vi "Periodic Tasks AUTO.vi"(8 "error in":errorcluster) -> ()   [LabVIEW 2013]
doc: "This VI runs in parallel to other tasks. It can contain as many user-defined periodic loops as you need. These can carry out PID or other sorts of timed response."
uses:
  <vilib>/Rock Robotics/SystemInterfaces/Utilities/FPGA_UtilitiesLED Source.ctl
  <vilib>/Rock Robotics/SystemInterfaces/Utilities/FPGA_UtilitiesLED State.ctl
  <vilib>/Rock Robotics/WPI/Relay/WPI_RelayValue.ctl
  <vilib>/Rock Robotics/WPI/DriverStation/DriverStationLCD/WPI_DriverStationLCDLCDLine.ctl
  <vilib>/Rock Robotics/WPI/Solenoid/WPI_SolenoidValue.ctl
  <vilib>/Rock Robotics/WPI/SafetyOutput/WPI_SafetyOutputConfigMenu.ctl
  Begin/Global Refnums.vi
  <vilib>/Rock Robotics/WPI/Solenoid/WPI_SolenoidSetEnum.vi
  <vilib>/Rock Robotics/WPI/Joystick/WPI_JoystickGetSetRefNum.vi
  <vilib>/Rock Robotics/WPI/Compressor/WPI_CompressorGetSetRefNum.vi
  Begin/Robot Global Data.vi
  Begin/Global Variables.vi
panel:
  out "Arm":string
  out "Shooter":string
  out "Winch":string
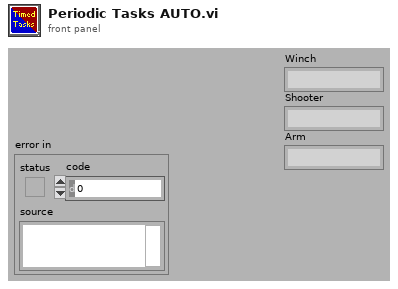
[diagram p1: front panel]
types:
  T1 = typedef "WPI_DriverStationLCDLCDLine.ctl" = enum16{"Main - Line 1", "User - Line 2", "User - Line 3", "User - Line 4", "User - Line 5", "User - Line 6"}
  T2 = typedef "WPI_CompressorDevRef.ctl" = cluster{"DevStatus":errorcluster, "DigitalInputDevRef":T3, "RelayDevRef":T6}
  T3 = typedef "WPI_DigitalInputDevRef.ctl" = cluster{"DevStatus":errorcluster, "DIO Channel":T4, "Digital Module":T5}
  T4 = typedef "FPGA_DIOChannel.ctl" = enum8{"DIO 1", "DIO 2", "DIO 3", "DIO 4", "DIO 5", "DIO 6", "DIO 7", "DIO 8", "DIO 9", "DIO 10", "DIO 11", "DIO 12", "DIO 13", "DIO 14", "Invalid"}
  T5 = typedef "FPGA_TypedefDigitalModule.ctl" = enum16{"Digital Module 1", "Digital Module 2"}
  T6 = typedef "WPI_RelayDevRef.ctl" = cluster{"DevStatus":errorcluster, "Relay Channel":T7, "Digital Module":T5, "Relay Direction":T8}
  T7 = typedef "FPGA_DIORelayChannel.ctl" = enum8{"Relay 1", "Relay 2", "Relay 3", "Relay 4", "Relay 5", "Relay 6", "Relay 7", "Relay 8", "Invalid"}
  T8 = typedef "WPI_RelayDirection.ctl" = enum16{"Both directions", "Forward only", "Reverse only"}
  T9 = typedef "WPI_RelayValue.ctl" = enum16{"Off", "On", "Forward", "Reverse"}
  T10 = typedef "WPI_SafetyOutputConfigMenu.ctl" = enum16{"Enable", "Disable"}
  T11 = typedef "WPI_SolenoidValue.ctl" = enum16{"Off", "On", "Forward", "Reverse"}
  T12 = typedef "WPI_SolenoidDevRef.ctl" = cluster{"DevStatus":errorcluster, "Solenoid Module":T13, "Forward Solenoid Channel":T14, "Reverse Solenoid Channel":T14}
  T13 = typedef "FPGA_TypedefSolenoidModule.ctl" = enum16{"Solenoid Module 1", "Solenoid Module 2"}
  T14 = typedef "WPI_SolenoidChannel.ctl" = enum8{"Solenoid 1", "Solenoid 2", "Solenoid 3", "Solenoid 4", "Solenoid 5", "Solenoid 6", "Solenoid 7", "Solenoid 8", "Invalid"}
  T15 = typedef "WPI_JoystickDevRef.ctl" = cluster{"Device":T16}
  T16 = typedef "WPI_JoystickDeviceEnum.ctl" = enum16{"USB 1", "USB 2", "USB 3", "USB 4", "Kinect 1", "Kinect 2"}
  T17 = typedef "WPI_JoystickButtonState.ctl" = cluster{"Button 1":bool, "Button 2":bool, "Button 3":bool, "Button 4":bool, "Button 5":bool, "Button 6":bool, "Button 7":bool, "Button 8":bool, "Button 9":bool, "Button 10":bool, "Button 11":bool, "Button 12":bool}
  T18 = typedef "WPI_EncoderDevRef.ctl" = cluster{"DevStatus":errorcluster, "EncoderIndex":T19, "CounterIndex":T20, "DistancePerCount":dbl, "Decoding Type":T21}
  T19 = typedef "FPGA_EncoderIdx.ctl" = enum8{"Enc 0", "Enc 1", "Enc 2", "Enc 3", "Invalid"}
  T20 = typedef "FPGA_CounterCtrSystemIndex.ctl" = enum8{"Ctr 0", "Ctr 1", "Ctr 2", "Ctr 3", "Ctr 4", "Ctr 5", "Ctr 6", "Ctr 7", "Invalid"}
  T21 = typedef "WPI_EncoderType.ctl" = enum16{"1x", "2x", "4x"}
  T22 = typedef "FPGA_UtilitiesLED State.ctl" = enum16{"Off", "On", "Toggle"}
  T23 = typedef "FPGA_UtilitiesLED Source.ctl" = enum16{"User LED", "FPGA LED"}
  T24 = typedef "WPI_MotorControlDeviceRef.ctl" = cluster{"DeviceStatus":errorcluster, "Type":enum16{"PWM", "CAN"}, "PWM":cluster{"Digital Module":T5, "PWM Channel":T25, "DeadBand":T26}, "CAN":cluster{"Device Number":u8, "Control Mode":T27, "Semaphore":T28, "Max Vout":dbl}, "Invert":bool, "TransformRef":T29, "InvTransformRef":T29}
  T25 = typedef "FPGA_DIOPWMChannel.ctl" = enum8{"PWM 1", "PWM 2", "PWM 3", "PWM 4", "PWM 5", "PWM 6", "PWM 7", "PWM 8", "PWM 9", "PWM 10", "Invalid"}
  T26 = typedef "WPI_PWMDeadband.ctl" = cluster{"Name":string, "maxPositivePwm":i32, "minPositivePwm":i32, "centerPwm":i32, "maxNegativePwm":i32, "minNegativePwm":i32, "angularRange":u16}
  T27 = typedef "WPI_CANJaguar_ControlMode.ctl" = enum8{"Percent VBus", "Current", "Speed", "Position", "Voltage"}
  T28 = typedef "Semaphore RefNum" = refnum<k1>
  T29 = typedef "WPI_PWMTransform_ConPane.ctl" = refnum<vi>
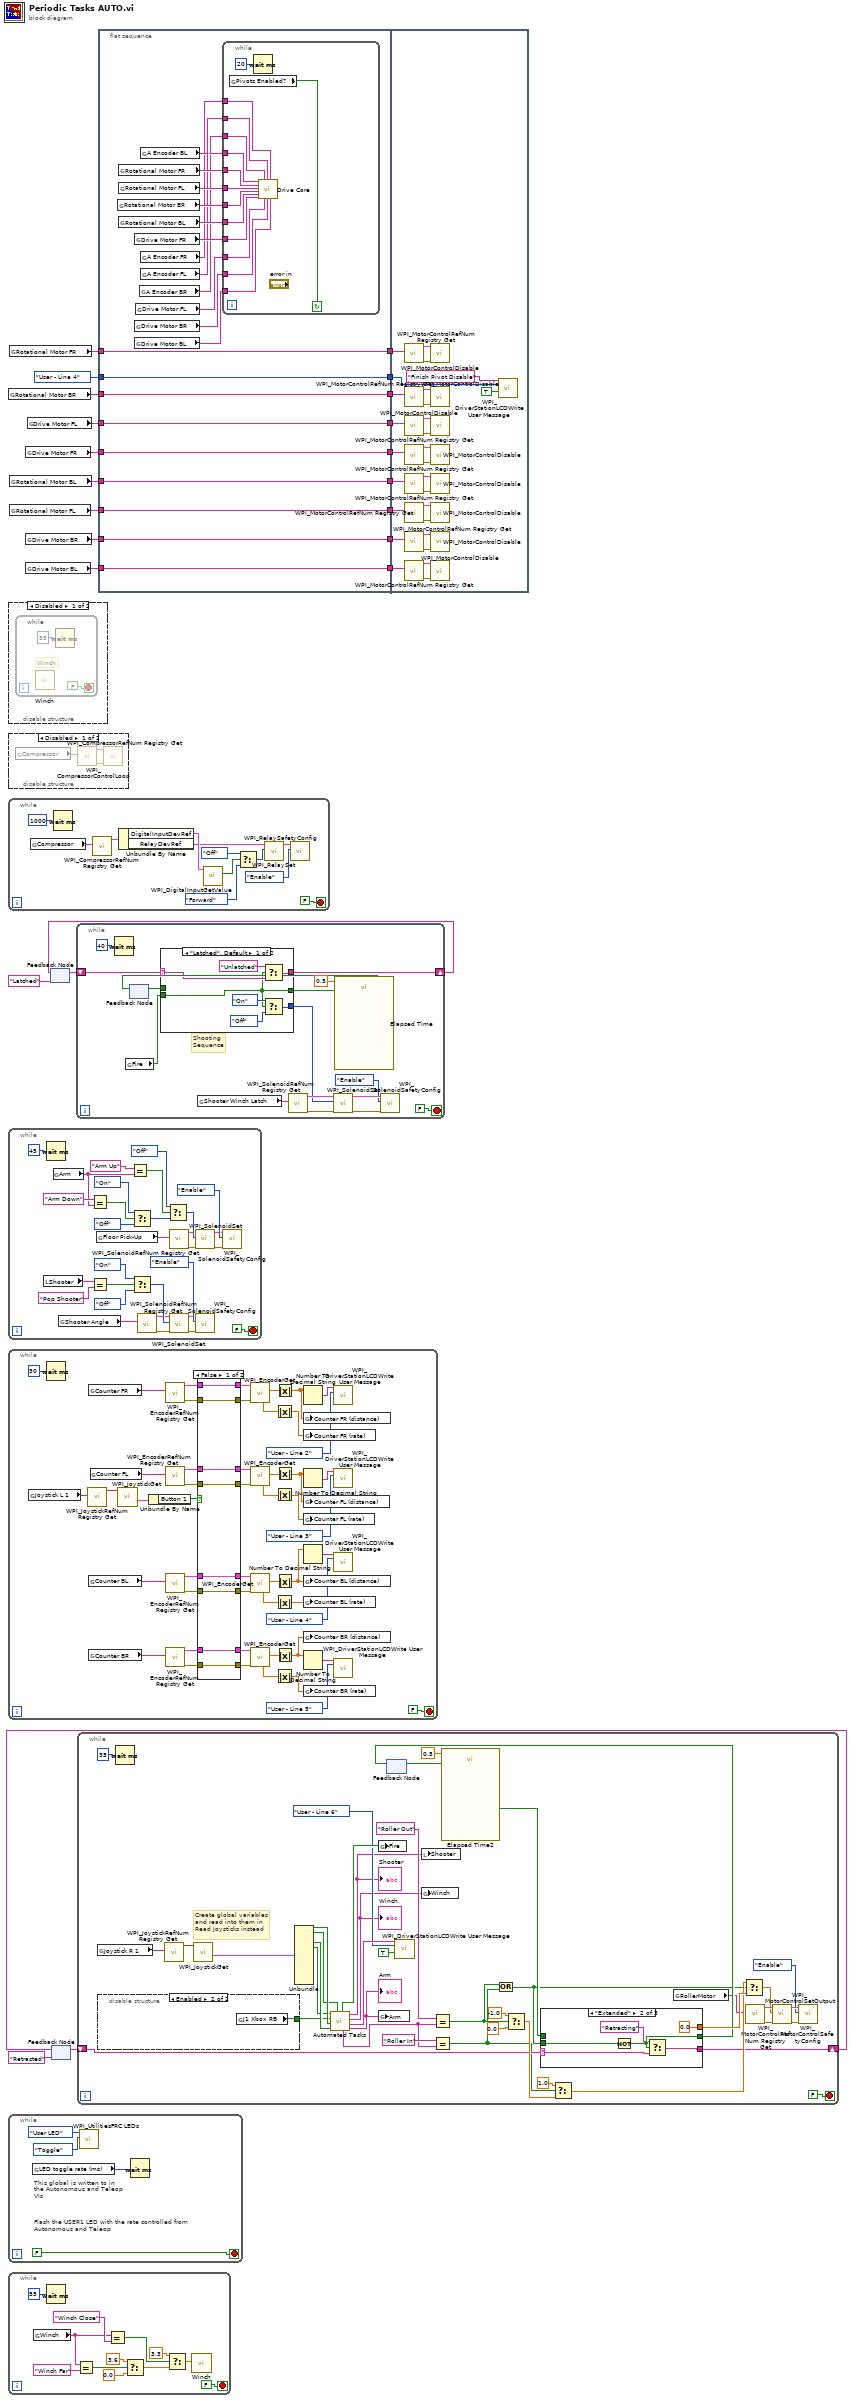
[diagram p0: block diagram]
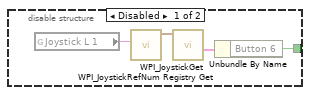
[diagram p3: hidden frame]
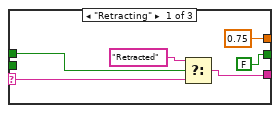
[diagram p4: hidden frame]
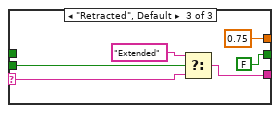
[diagram p5: hidden frame]
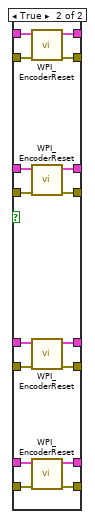
[diagram p6: hidden frame]
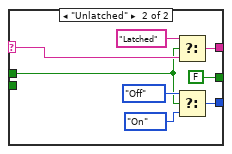
[diagram p7: hidden frame]
diagram:
  n1 = global read "Global Refnums.vi" "Rotational Motor BR"() -> (w22:string)
  n2 = disable-structure shown="Disabled" {
    frame Disabled {
      n3 = while {
        stop <- FALSE stop-if-true
        # "Winch"
        n4 = call "Winch.vi"() -> ()  [unwired: 12 in]
        n5 = Wait (ms)(milliseconds to wait=u32 35) -> ()  [unwired: 1 out]
      }
    }
    frame Enabled {
    }
  }
  n6 = disable-structure shown="Disabled" {
    frame Disabled {
      n7 = global read "Global Refnums.vi" "Compressor"() -> (w29:string)
      n8 = call <vilib>:"WPI_CompressorRefNum Registry Get.vi"("refnum name"=w29) -> ("error out"=w28:errorcluster, "CompressorDevRef"=w27:T2)  [unwired: 9 in]
      n9 = call <vilib>:"WPI_CompressorControlLoop.vi"("error in (no error)"=w28, "CompressorDevRef"=w27) -> ()  [unwired: 10 in]
    }
    frame Enabled {
    }
  }
  n10 = while {
    stop <- FALSE stop-if-true
    n11 = global read "Global Refnums.vi" "Compressor"() -> (w39:string)
    n12 = Wait (ms)(milliseconds to wait=1000) -> ()  [unwired: 1 out]
    n13 = call <vilib>:"WPI_CompressorRefNum Registry Get.vi"("refnum name"=w39) -> ("CompressorDevRef"=w38:T2)  [unwired: 9 in, 1 out]
    n14 = Unbundle By Name(w38) -> ("DigitalInputDevRef"=w37:T3, "RelayDevRef"=w36:T6)
    n15 = call <vilib>:"WPI_DigitalInputGetValue.vi"("DigitalInputDevRef"=w37) -> ("Value"=w33:bool)  [unwired: 8 in, 2 out]
    n16 = Select(t=WPI_RelayValue."Off" ("RelayValue"), s=w33, f=WPI_RelayValue."Forward" ("RelayValue")) -> (s? t:f=w32:T9)
    n17 = call <vilib>:"WPI_RelaySet.vi"("RelayValue"=w32, "RelayDevRef"=w36) -> ("RelayDevRef"=w35:T6)  [unwired: 8 in, 1 out]
    n18 = call <vilib>:"WPI_RelaySafetyConfig.vi"("mode"=WPI_SafetyOutputConfigMenu."Enable", "RelayDevRef"=w35) -> ()  [unwired: 8 in, 2 out]
  }
  n19 = while {
    stop <- FALSE stop-if-true
    n20 = local read "Shooter"() -> (w59:string)
    n21 = Wait (ms)(milliseconds to wait=u32 45) -> ()  [unwired: 1 out]
    n22 = global read "Global Refnums.vi" "Arm"() -> (w42:string)
    n23 = global read "Global Refnums.vi" "Shooter Angle"() -> (w70:string)
    n24 = Equal?(x="Arm Down", y=w42) -> (x = y?=w44:bool)
    n25 = Equal?(x=w59, y="Pop Shooter") -> (x = y?=w60:bool)
    n26 = global read "Global Refnums.vi" "Floor Pick-Up"() -> (w54:string)
    n27 = Equal?(x="Arm Up", y=w42) -> (x = y?=w56:bool)
    n28 = Select(t=WPI_SolenoidValue."On" ("Value"), s=w44, f=WPI_SolenoidValue."Off" ("Value")) -> (s? t:f=w43:T11)
    n29 = Select(t=WPI_SolenoidValue."On" ("Value"), s=w60, f=WPI_SolenoidValue."Off" ("Value")) -> (s? t:f=w69:T11)
    n30 = call <vilib>:"WPI_SolenoidRefNum Registry Get.vi"("refnum name"=w70) -> ("error out"=w62:errorcluster, "SolenoidDevRef"=w63:T12)  [unwired: 9 in]
    n31 = Select(t=WPI_SolenoidValue."Off" ("Value"), s=w56, f=w43) -> (s? t:f=w57:T11)
    n32 = call <vilib>:"WPI_SolenoidRefNum Registry Get.vi"("refnum name"=w54) -> ("error out"=w49:errorcluster, "SolenoidDevRef"=w50:T12)  [unwired: 9 in]
    n33 = call-poly <vilib>:"WPI_SolenoidSet.vi"("error in (no error)"=w62, "Value"=w69, "SolenoidDevRef"=w63) -> ("error out"=w65:errorcluster, "SolenoidDevRef"=w64:T12)  [unwired: 7 in]
    n34 = call-poly <vilib>:"WPI_SolenoidSet.vi"("error in (no error)"=w49, "Value"=w57, "SolenoidDevRef"=w50) -> ("error out"=w52:errorcluster, "SolenoidDevRef"=w51:T12)  [unwired: 7 in]
    n35 = call <vilib>:"WPI_SolenoidSafetyConfig.vi"("error in (no error)"=w65, "mode"=WPI_SafetyOutputConfigMenu."Enable", "SolenoidDevRef"=w64) -> ()  [unwired: 7 in, 2 out]
    n36 = call <vilib>:"WPI_SolenoidSafetyConfig.vi"("error in (no error)"=w52, "mode"=WPI_SafetyOutputConfigMenu."Enable", "SolenoidDevRef"=w51) -> ()  [unwired: 7 in, 2 out]
  }
  n37 = while {
    stop <- FALSE stop-if-true
    n38 = global read "Global Refnums.vi" "Joystick L 1"() -> (w118:string)
    n39 = Wait (ms)(milliseconds to wait=u32 30) -> ()  [unwired: 1 out]
    n40 = call <vilib>:"WPI_JoystickRefNum Registry Get.vi"("refnum name"=w118) -> ("JoystickDevRef"=w119:T15)  [unwired: 9 in, 1 out]
    n41 = global read "Global Refnums.vi" "Counter FR"() -> (w82:string)
    n42 = global read "Global Refnums.vi" "Counter BL"() -> (w83:string)
    n43 = global read "Global Refnums.vi" "Counter BR"() -> (w80:string)
    n44 = global read "Global Refnums.vi" "Counter FL"() -> (w81:string)
    n45 = call <vilib>:"WPI_JoystickGet.vi"("JoystickDevRef"=w119) -> ("Buttons"=w117:T17)  [unwired: 4 in, 2 out]
    n46 = Unbundle By Name(w117) -> ("Button 1"=w116:bool)
    n47 = call <vilib>:"WPI_EncoderRefNum Registry Get.vi"("refnum name"=w82) -> ("error out"=w100:errorcluster, "EncoderDevRef"=w103:T18)  [unwired: 9 in]
    n48 = call <vilib>:"WPI_EncoderRefNum Registry Get.vi"("refnum name"=w81) -> ("error out"=w105:errorcluster, "EncoderDevRef"=w106:T18)  [unwired: 9 in]
    n49 = call <vilib>:"WPI_EncoderRefNum Registry Get.vi"("refnum name"=w83) -> ("error out"=w110:errorcluster, "EncoderDevRef"=w111:T18)  [unwired: 9 in]
    n50 = call <vilib>:"WPI_EncoderRefNum Registry Get.vi"("refnum name"=w80) -> ("error out"=w108:errorcluster, "EncoderDevRef"=w109:T18)  [unwired: 9 in]
    n51 = case shown="False" w116 {
      tunnel: w109 -> [w126 w145]
      tunnel: [w126 w144] -> w114
      tunnel: [w128 w143] -> w115
      tunnel: w108 -> [w128 w142]
      tunnel: [w127 w141] -> w113
      tunnel: [w129 w140] -> w112
      tunnel: w111 -> [w127 w139]
      tunnel: w110 -> [w129 w138]
      tunnel: [w125 w130] -> w107
      tunnel: w106 -> [w125 w137]
      tunnel: w105 -> [w124 w136]
      tunnel: [w124 w131] -> w104
      tunnel: w103 -> [w123 w135]
      tunnel: [w123 w132] -> w102
      tunnel: [w122 w133] -> w101
      tunnel: w100 -> [w122 w134]
      frame False {
      }
      frame True {
        n52 = call <vilib>:"WPI_EncoderReset.vi"("error in (no error)"=w134, "EncoderDevRef"=w135) -> ("error out"=w133:errorcluster, "EncoderDevRef"=w132:T18)  [unwired: 8 in]
        n53 = call <vilib>:"WPI_EncoderReset.vi"("error in (no error)"=w136, "EncoderDevRef"=w137) -> ("error out"=w131:errorcluster, "EncoderDevRef"=w130:T18)  [unwired: 8 in]
        n54 = call <vilib>:"WPI_EncoderReset.vi"("error in (no error)"=w138, "EncoderDevRef"=w139) -> ("error out"=w140:errorcluster, "EncoderDevRef"=w141:T18)  [unwired: 8 in]
        n55 = call <vilib>:"WPI_EncoderReset.vi"("error in (no error)"=w142, "EncoderDevRef"=w145) -> ("error out"=w143:errorcluster, "EncoderDevRef"=w144:T18)  [unwired: 8 in]
      }
    }
    n56 = call <vilib>:"WPI_EncoderGet.vi"("error in (no error)"=w101, "EncoderDevRef"=w102) -> ("Distance"=w97:dbl, "Rate"=w93:dbl)  [unwired: 4 in, 4 out]
    n57 = call <vilib>:"WPI_EncoderGet.vi"("error in (no error)"=w104, "EncoderDevRef"=w107) -> ("Distance"=w99:dbl, "Rate"=w95:dbl)  [unwired: 4 in, 4 out]
    n58 = call <vilib>:"WPI_EncoderGet.vi"("error in (no error)"=w112, "EncoderDevRef"=w113) -> ("Distance"=w98:dbl, "Rate"=w94:dbl)  [unwired: 4 in, 4 out]
    n59 = call <vilib>:"WPI_EncoderGet.vi"("error in (no error)"=w115, "EncoderDevRef"=w114) -> ("Distance"=w96:dbl, "Rate"=w92:dbl)  [unwired: 4 in, 4 out]
    n60 = Absolute Value(x=w93) -> (abs(x)=w78:dbl)
    n61 = Absolute Value(x=w95) -> (abs(x)=w76:dbl)
    n62 = Absolute Value(x=w94) -> (abs(x)=w74:dbl)
    n63 = Absolute Value(x=w92) -> (abs(x)=w72:dbl)
    n64 = Absolute Value(x=w97) -> (abs(x)=w79:dbl)
    n65 = Absolute Value(x=w99) -> (abs(x)=w77:dbl)
    n66 = Absolute Value(x=w98) -> (abs(x)=w75:dbl)
    n67 = Absolute Value(x=w96) -> (abs(x)=w73:dbl)
    n68 = Number To Decimal String(number=w79) -> (decimal integer string=w90:string)  [unwired: 1 in]
    n69 = global write "Global Refnums.vi" "Counter FR (distance)"(w79) -> ()
    n70 = global write "Global Refnums.vi" "Counter FR (rate)"(w78) -> ()
    n71 = Number To Decimal String(number=w77) -> (decimal integer string=w89:string)  [unwired: 1 in]
    n72 = global write "Global Refnums.vi" "Counter FL (distance)"(w77) -> ()
    n73 = global write "Global Refnums.vi" "Counter FL (rate)"(w76) -> ()
    n74 = Number To Decimal String(number=w75) -> (decimal integer string=w88:string)  [unwired: 1 in]
    n75 = global write "Global Refnums.vi" "Counter BL (distance)"(w75) -> ()
    n76 = global write "Global Refnums.vi" "Counter BL (rate)"(w74) -> ()
    n77 = global write "Global Refnums.vi" "Counter BR (distance)"(w73) -> ()
    n78 = Number To Decimal String(number=w73) -> (decimal integer string=w91:string)  [unwired: 1 in]
    n79 = global write "Global Refnums.vi" "Counter BR (rate)"(w72) -> ()
    n80 = call <vilib>:"WPI_DriverStationLCDWrite User Message.vi"("line text"=w90, "line"=WPI_DriverStationLCDLCDLine."User - Line 2") -> ()  [unwired: 13 in, 1 out]
    n81 = call <vilib>:"WPI_DriverStationLCDWrite User Message.vi"("line text"=w89, "line"=WPI_DriverStationLCDLCDLine."User - Line 3") -> ()  [unwired: 13 in, 1 out]
    n82 = call <vilib>:"WPI_DriverStationLCDWrite User Message.vi"("line text"=w88, "line"=WPI_DriverStationLCDLCDLine."User - Line 4") -> ()  [unwired: 13 in, 1 out]
    n83 = call <vilib>:"WPI_DriverStationLCDWrite User Message.vi"("line text"=w91, "line"=WPI_DriverStationLCDLCDLine."User - Line 5") -> ()  [unwired: 13 in, 1 out]
  }
  n84 = while {
    stop <- FALSE stop-if-true
    # "This global is written to in the Autonomous and Teleop VIs"
    # "Flash the USER1 LED with the rate controlled from Autonomous and Teleop"
    n85 = global read "Robot Global Data.vi" "LED toggle rate (ms)"() -> (w146:u32)
    n86 = call <vilib>:"WPI_UtilitiesFRC LEDs.vi"("State"=FPGA_UtilitiesLED_State."Toggle", "LED Type"=FPGA_UtilitiesLED_Source."User LED") -> ()  [unwired: 1 in, 9 out]
    n87 = Wait (ms)(milliseconds to wait=w146) -> ()  [unwired: 1 out]
  }
  n88 = while {
    stop <- FALSE stop-if-true
    n89 = global read "Global Refnums.vi" "Winch"() -> (w150:string)
    n90 = Wait (ms)(milliseconds to wait=u32 55) -> ()  [unwired: 1 out]
    n91 = Equal?(x=w150, y="Winch Far") -> (x = y?=w156:bool)
    n92 = Equal?(x=w150, y="Winch Close") -> (x = y?=w154:bool)
    n93 = Select(t=3.6, s=w156, f=0.0) -> (s? t:f=w158:dbl)
    n94 = Select(t=3.3, s=w154, f=w158) -> (s? t:f=w159:dbl)
    n95 = call "Winch.vi"("setpoint"=w159) -> ()  [unwired: 11 in]
  }
  n96 = global read "Global Refnums.vi" "Rotational Motor FR"() -> (w24:string)
  n97 = global read "Global Refnums.vi" "Rotational Motor BL"() -> (w21:string)
  n98 = global read "Global Refnums.vi" "Rotational Motor FL"() -> (w23:string)
  n99 = global read "Global Refnums.vi" "Drive Motor FR"() -> (w20:string)
  n100 = global read "Global Refnums.vi" "Drive Motor BR"() -> (w18:string)
  n101 = global read "Global Refnums.vi" "Drive Motor BL"() -> (w17:string)
  n102 = global read "Global Refnums.vi" "Drive Motor FL"() -> (w19:string)
  n103 = feedback #1("Latched") -> (w5:string)
  n104 = feedback #2("Retracted") -> (w2:string)
  n105 = while {
    shift-right: [w171] -> w6
    shift-left: w5 -> [w170]
    stop <- FALSE stop-if-true
    # "Shooting\nSequence"
    n106 = Wait (ms)(milliseconds to wait=u32 40) -> ()  [unwired: 1 out]
    n107 = global read "Global Variables.vi" "Fire"() -> (w169:bool)
    n108 = feedback #3() -> (w165:bool)  [unwired: 1 in]
    n109 = case shown="\"Latched\", Default" w170 {
      selector: w170 -> [w183 w191]
      tunnel: [w182 w190] -> w171
      tunnel: w169 -> [w178 _]
      tunnel: [w179 w187] -> w168
      tunnel: [w178 FALSE] -> w167
      tunnel: w165 -> [_ w186]
      frame "Latched", Default {
        n110 = Select(t="Unlatched", s=w178, f=w183) -> (s? t:f=w182:string)
        n111 = Select(t=WPI_SolenoidValue."On" ("Value"), s=w178, f=WPI_SolenoidValue."Off" ("Value")) -> (s? t:f=w179:T11)
      }
      frame "Unlatched" {
        n112 = Select(t="Latched", s=w186, f=w191) -> (s? t:f=w190:string)
        n113 = Select(t=WPI_SolenoidValue."Off" ("Value"), s=w186, f=WPI_SolenoidValue."On" ("Value")) -> (s? t:f=w187:T11)
      }
    }
    n114 = global read "Global Refnums.vi" "Shooter Winch Latch"() -> (w177:string)
    n115 = call <vilib>:"WPI_SolenoidRefNum Registry Get.vi"("refnum name"=w177) -> ("error out"=w176:errorcluster, "SolenoidDevRef"=w175:T12)  [unwired: 9 in]
    n116 = call-poly <vilib>:"WPI_SolenoidSet.vi"("error in (no error)"=w176, "Value"=w168, "SolenoidDevRef"=w175) -> ("error out"=w174:errorcluster, "SolenoidDevRef"=w173:T12)  [unwired: 7 in]
    n117 = call "Elapsed Time"("Time Target (s)"=0.5, "Reset"=w167) -> ("Time has Elapsed"=w166:bool)  [unwired: 10 in, 7 out]
    n118 = feedback-in #3(w166) -> ()
    n119 = call <vilib>:"WPI_SolenoidSafetyConfig.vi"("error in (no error)"=w174, "mode"=WPI_SafetyOutputConfigMenu."Enable", "SolenoidDevRef"=w173) -> ()  [unwired: 7 in, 2 out]
  }
  n120 = feedback-in #1(w6) -> ()
  n121 = while {
    shift-right: [w220] -> w1
    shift-left: w2 -> [w218]
    stop <- FALSE stop-if-true
    # "Create global variables\nand read into them in \nRead Joysticks instead"
    n122 = global read "Global Refnums.vi" "Joystick R 1"() -> (w214:string)
    n123 = disable-structure shown="Enabled" {
      disable-tunnel: [w235 w239] -> w208
      frame Disabled {
        n124 = global read "Global Refnums.vi" "Joystick L 1"() -> (w237:string)
        n125 = call <vilib>:"WPI_JoystickRefNum Registry Get.vi"("refnum name"=w237) -> ("JoystickDevRef"=w238:T15)  [unwired: 9 in, 1 out]
        n126 = call <vilib>:"WPI_JoystickGet.vi"("JoystickDevRef"=w238) -> ("Buttons"=w236:T17)  [unwired: 4 in, 2 out]
        n127 = Unbundle By Name(w236) -> ("Button 6"=w235:bool)
      }
      frame Enabled {
        n128 = global read "Global Variables.vi" "J1 Xbox RB"() -> (w239:bool)
      }
    }
    n129 = Wait (ms)(milliseconds to wait=u32 35) -> ()  [unwired: 1 out]
    n130 = call <vilib>:"WPI_JoystickRefNum Registry Get.vi"("refnum name"=w214) -> ("JoystickDevRef"=w234:T15)  [unwired: 9 in, 1 out]
    n131 = call <vilib>:"WPI_JoystickGet.vi"("JoystickDevRef"=w234) -> ("Buttons"=w233:T17)  [unwired: 4 in, 2 out]
    n132 = Unbundle(w233) -> ("Button 1"=w212:bool, "Button 2"=w211:bool, "Button 4"=w210:bool, "Button 5"=w209:bool)  [unwired: 8 out]
    n133 = call "Automated Tasks.vi"("RB"=w209, "Fire"=w208, "A"=w212, "Y"=w210, "B"=w211) -> ("Fire"=w204:bool, "Roller"=w199:string, "Shooter"=w195:string, "Winch"=w193:string, "Case"=w203:string, "Arm"=w194:string)
    "Winch" <- w193
    "Shooter" <- w195
    "Arm" <- w194
    n134 = global write "Global Variables.vi" "Fire"(w204) -> ()
    n135 = global write "Global Refnums.vi" "Arm"(w194) -> ()
    n136 = feedback #4() -> (w216:bool)  [unwired: 1 in]
    n137 = call <vilib>:"WPI_DriverStationLCDWrite User Message.vi"("line text"=w203, "line"=WPI_DriverStationLCDLCDLine."User - Line 6", "clear line before write (T)"=TRUE) -> ()  [unwired: 12 in, 1 out]
    n138 = local write "Shooter"(w195) -> ()
    n139 = global write "Global Refnums.vi" "Winch"(w193) -> ()
    n140 = Equal?(x="Roller Out", y=w199) -> (x = y?=w198:bool)
    n141 = Equal?(x="Roller In", y=w199) -> (x = y?=w197:bool)
    n142 = call "Elapsed Time2"("Time Target (s)"=0.5, "Reset"=w216) -> ("Time has Elapsed"=w200:bool)  [unwired: 10 in, 7 out]
    n143 = Or(x=w198, y=w197) -> (x .or. y?=w196:bool)
    n144 = Select(t=-1.0, s=w198, f=0.0) -> (s? t:f=w224:dbl)
    n145 = case shown="\"Extended\"" w218 {
      selector: w218 -> [w244 w246 w255]
      tunnel: [0.75 0.0 0.75] -> w222
      tunnel: w196 -> [_ w249 w253]
      tunnel: [w243 w250 w254] -> w220
      tunnel: w200 -> [w242 _ _]
      tunnel: [FALSE w248 FALSE] -> w217
      frame "Retracting" {
        n146 = Select(t="Retracted", s=w242, f=w244) -> (s? t:f=w243:string)
      }
      frame "Extended" {
        n147 = Not(x=w249) -> (.not. x?=w248:bool)
        n148 = Select(t="Retracting" ("f"), s=w248, f=w246) -> (s? t:f=w250:string)
      }
      frame "Retracted", Default {
        n149 = Select(t="Extended", s=w253, f=w255) -> (s? t:f=w254:string)
      }
    }
    n150 = feedback-in #4(w217) -> ()
    n151 = Select(t=1.0, s=w197, f=w224) -> (s? t:f=w221:dbl)
    n152 = global read "Global Refnums.vi" "RollerMotor"() -> (w207:string)
    n153 = Select(t=w221, s=w196, f=w222) -> (s? t:f=w223:dbl)
    n154 = call <vilib>:"WPI_MotorControlRefNum Registry Get.vi"("refnum name"=w207) -> ("error out"=w230:errorcluster, "MotorControlDevRef"=w232:T24)  [unwired: 9 in]
    n155 = call <vilib>:"WPI_MotorControlSetOutput.vi"("error in (no error)"=w230, "Output"=w223, "MotorControlDevRef"=w232) -> ("error out"=w229:errorcluster, "MotorControlDevRef"=w231:T24)  [unwired: 6 in, 1 out]
    n156 = call <vilib>:"WPI_MotorControlSafetyConfig.vi"("error in (no error)"=w229, "mode"=WPI_SafetyOutputConfigMenu."Enable", "MotorControlDevRef"=w231) -> ()  [unwired: 7 in, 2 out]
  }
  n157 = feedback-in #2(w1) -> ()
  n158 = flat-sequence {
    tunnel: WPI_DriverStationLCDLCDLine."User - Line 4" ("line") -> [w270]
    tunnel: w19 -> [w271]
    tunnel: w17 -> [w272]
    tunnel: w18 -> [w273]
    tunnel: w20 -> [w274]
    tunnel: w21 -> [w275]
    tunnel: w22 -> [w276]
    tunnel: w23 -> [w277]
    tunnel: w24 -> [w278]
    tunnel: [w278] -> w15
    tunnel: [w277] -> w14
    tunnel: [w276] -> w13
    tunnel: [w275] -> w12
    tunnel: [w274] -> w11
    tunnel: [w273] -> w10
    tunnel: [w272] -> w9
    tunnel: [w271] -> w8
    tunnel: [w270] -> w7
    tunnel: w15 -> [w319]
    tunnel: w14 -> [w312]
    tunnel: w13 -> [w311]
    tunnel: w12 -> [w308]
    tunnel: w11 -> [w299]
    tunnel: w10 -> [w298]
    tunnel: w9 -> [w297]
    tunnel: w8 -> [w296]
    tunnel: w7 -> [w295]
    frame #0 {
      n159 = global read "Global Refnums.vi" "Rotational Motor BR"() -> (w264:string)
      n160 = global read "Global Refnums.vi" "Rotational Motor FR"() -> (w262:string)
      n161 = global read "Global Refnums.vi" "Rotational Motor FL"() -> (w263:string)
      n162 = global read "Global Refnums.vi" "Rotational Motor BL"() -> (w265:string)
      n163 = global read "Global Refnums.vi" "Drive Motor FR"() -> (w266:string)
      n164 = global read "Global Refnums.vi" "Drive Motor BR"() -> (w268:string)
      n165 = global read "Global Refnums.vi" "Drive Motor BL"() -> (w269:string)
      n166 = global read "Global Refnums.vi" "Drive Motor FL"() -> (w267:string)
      n167 = global read "Global Refnums.vi" "A Encoder BR"() -> (w259:string)
      n168 = global read "Global Refnums.vi" "A Encoder BL"() -> (w260:string)
      n169 = global read "Global Refnums.vi" "A Encoder FR"() -> (w258:string)
      n170 = global read "Global Refnums.vi" "A Encoder FL"() -> (w261:string)
      n171 = while {
        tunnel: w258 -> [w292]
        tunnel: w259 -> [w290]
        tunnel: w260 -> [w289]
        tunnel: w261 -> [w291]
        tunnel: w266 -> [w284]
        tunnel: w268 -> [w282]
        tunnel: w269 -> [w281]
        tunnel: w267 -> [w283]
        tunnel: w262 -> [w288]
        tunnel: w264 -> [w286]
        tunnel: w265 -> [w285]
        tunnel: w263 -> [w287]
        stop <- w279 continue-if-true
        n172 = global read "Global Variables.vi" "Pivots Enabled?"() -> (w279:bool)
        n173 = Wait (ms)(milliseconds to wait=u32 20) -> ()  [unwired: 1 out]
        n174 = call "Drive Core.vi"("A Encoder BL"=w289, "Rotational Motor FR"=w288, "Rotational Motor FL"=w287, "Rotational Motor BR"=w286, "Rotational Motor BL"=w285, "Drive Motor FR"=w284, "A Encoder BR"=w290, "Drive Motor FL"=w283, "A Encoder FL"=w291, "Drive Motor BR"=w282, "A Encoder FR"=w292, "Drive Motor BL"=w281) -> ()  [unwired: 8 in]
      }
    }
    frame #1 {
      n175 = call <vilib>:"WPI_MotorControlRefNum Registry Get.vi"("refnum name"=w319) -> ("error out"=w317:errorcluster, "MotorControlDevRef"=w318:T24)  [unwired: 9 in]
      n176 = call <vilib>:"WPI_MotorControlRefNum Registry Get.vi"("refnum name"=w311) -> ("error out"=w313:errorcluster, "MotorControlDevRef"=w314:T24)  [unwired: 9 in]
      n177 = call <vilib>:"WPI_MotorControlRefNum Registry Get.vi"("refnum name"=w296) -> ("error out"=w303:errorcluster, "MotorControlDevRef"=w302:T24)  [unwired: 9 in]
      n178 = call <vilib>:"WPI_MotorControlRefNum Registry Get.vi"("refnum name"=w299) -> ("error out"=w301:errorcluster, "MotorControlDevRef"=w300:T24)  [unwired: 9 in]
      n179 = call <vilib>:"WPI_MotorControlRefNum Registry Get.vi"("refnum name"=w308) -> ("error out"=w309:errorcluster, "MotorControlDevRef"=w310:T24)  [unwired: 9 in]
      n180 = call <vilib>:"WPI_MotorControlRefNum Registry Get.vi"("refnum name"=w312) -> ("error out"=w315:errorcluster, "MotorControlDevRef"=w316:T24)  [unwired: 9 in]
      n181 = call <vilib>:"WPI_MotorControlRefNum Registry Get.vi"("refnum name"=w298) -> ("error out"=w305:errorcluster, "MotorControlDevRef"=w304:T24)  [unwired: 9 in]
      n182 = call <vilib>:"WPI_MotorControlRefNum Registry Get.vi"("refnum name"=w297) -> ("error out"=w307:errorcluster, "MotorControlDevRef"=w306:T24)  [unwired: 9 in]
      n183 = call <vilib>:"WPI_MotorControlDisable.vi"("error in (no error)"=w317, "MotorControlDevRef"=w318) -> ()  [unwired: 8 in, 2 out]
      n184 = call <vilib>:"WPI_MotorControlDisable.vi"("error in (no error)"=w313, "MotorControlDevRef"=w314) -> ()  [unwired: 8 in, 2 out]
      n185 = call <vilib>:"WPI_MotorControlDisable.vi"("error in (no error)"=w303, "MotorControlDevRef"=w302) -> ()  [unwired: 8 in, 2 out]
      n186 = call <vilib>:"WPI_MotorControlDisable.vi"("error in (no error)"=w301, "MotorControlDevRef"=w300) -> ()  [unwired: 8 in, 2 out]
      n187 = call <vilib>:"WPI_MotorControlDisable.vi"("error in (no error)"=w309, "MotorControlDevRef"=w310) -> ()  [unwired: 8 in, 2 out]
      n188 = call <vilib>:"WPI_MotorControlDisable.vi"("error in (no error)"=w315, "MotorControlDevRef"=w316) -> ()  [unwired: 8 in, 2 out]
      n189 = call <vilib>:"WPI_MotorControlDisable.vi"("error in (no error)"=w305, "MotorControlDevRef"=w304) -> ()  [unwired: 8 in, 2 out]
      n190 = call <vilib>:"WPI_MotorControlDisable.vi"("error in (no error)"=w307, "MotorControlDevRef"=w306) -> ()  [unwired: 8 in, 2 out]
      n191 = call <vilib>:"WPI_DriverStationLCDWrite User Message.vi"("line text"="Finish Pivot Disable", "line"=w295, "clear line before write (T)"=TRUE) -> ()  [unwired: 12 in, 1 out]
    }
  }
